vi "asdk Set.vi"(8 "error in (no error)":errorcluster, 9 "value":dbl, 10 "command":string, 11 "pDm":u32) -> (0 "error out":errorcluster, 3 "pDm out":u32)   [LabVIEW 2019, in "ASDK.lvlib"]
doc: "ASDK_API COMPL_STAT asdkSet( asdkDM *pDm, CStrConst command, Scalar value );"
uses:
  <userlib>/asdk.lib/ASDK.lvlib
  ASDK.dll
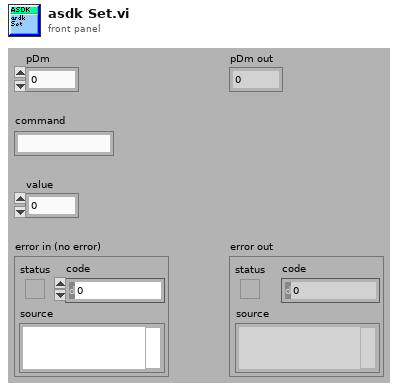
[diagram p1: front panel]
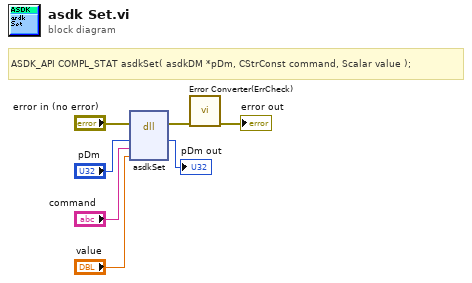
[diagram p0: block diagram]
diagram:
  # "ASDK_API COMPL_STAT asdkSet( asdkDM *pDm, CStrConst command, Scalar value );"
  n1 = dll-call lib="ASDK.*" fn="asdkSet"(error in="error in (no error)", "pDm"="pDm", "command"="command", "value"="value") -> (error out=w2:errorcluster, "pDm"=→"pDm out":u32)  [unwired: 5 in, 1 out]
  n2 = call <userlib>:"Error Converter(ErrCheck).vi"("error in (no error)"=w2) -> ("error out"=→"error out":errorcluster)  [unwired: 10 in]
